vi "Sensor Read 2017.vi"() -> ()   [LabVIEW 2016]
uses:
  Global Variables/Refnum Names.vi
  Global Variables/Sensor Data.vi
panel:
  out "YPR.Yaw":dbl
  out "FusedHeading.Heading":dbl
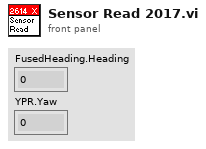
[diagram p1: front panel]
types:
  T1 = typedef "WPI_MotorControlDeviceRef.ctl" = cluster{"DeviceStatus":errorcluster, "Type":T2, "PWM":cluster{"PWM Channel":T3, "DeadBand":T4}, "CAN":cluster{"Device Number":u8, "SetOutput VI Ref":variant, "GetOutput VI Ref":variant, "Enable VI Ref":variant, "Disable VI Ref":variant, "Data":variant}, "Invert":bool}
  T2 = typedef "WPI_MotorControlType.ctl" = enum16{"PWM", "CAN"}
  T3 = typedef "FPGA_DIOPWMChannel.ctl" = enum8{"PWM 0", "PWM 1", "PWM 2", "PWM 3", "PWM 4", "PWM 5", "PWM 6", "PWM 7", "PWM 8", "PWM 9", "PWM MXP 0", "PWM MXP 1", "PWM MXP 2", "PWM MXP 3", "PWM MXP 4", "PWM MXP 5", "PWM MXP 6", "PWM MXP 7", "PWM MXP 8", "PWM MXP 9", "Invalid"}
  T4 = typedef "WPI_PWMDeadband.ctl" = cluster{"Name":string, "maxPositivePwm":i32, "minPositivePwm":i32, "centerPwm":i32, "maxNegativePwm":i32, "minNegativePwm":i32, "angularRange":u16}
  T5 = typedef "CTRE_PigeonIMU_DeviceRef.ctl" = cluster{"DeviceStatus":errorcluster, "Device Number":u8, "Type":T6, "Device ID":u32}
  T6 = typedef "CTRE_PigeonIMU_ConnectionType.ctl" = u32
  T7 = typedef "WPI_DigitalInputDevRef.ctl" = cluster{"DevStatus":errorcluster, "DIO Channel":T8}
  T8 = typedef "FPGA_DIOChannel.ctl" = enum8{"DIO 0", "DIO 1", "DIO 2", "DIO 3", "DIO 4", "DIO 5", "DIO 6", "DIO 7", "DIO 8", "DIO 9", "DIO MXP 0", "DIO MXP 1", "DIO MXP 2", "DIO MXP 3", "DIO MXP 4", "DIO MXP 5", "DIO MXP 6", "DIO MXP 7", "DIO MXP 8", "DIO MXP 9", "DIO MXP 10", "DIO MXP 11", "DIO MXP 12", "DIO MXP 13", "DIO MXP 14", "DIO MXP 15", "SPI Port CS1", "SPI Port CS2", "SPI Port CS3", "SPI Port MISO", "SPI Port MOSI", "Invalid"}
  T9 = typedef "CTRE_PigeonIMU_GlobalStatus.ctl" = cluster{"PigeonState":T10, "FusedHeading":cluster{"Heading":dbl, "Valid?":bool, "Fusing?":bool}, "YPR":cluster{"Yaw":dbl, "Pitch":dbl, "Roll":dbl}, "Compass":cluster{"Heading":dbl, "Magnitude":dbl, "Absolute Heading":dbl}, "Accelerometer":cluster{"Biased":cluster{"X":i16, "Y":i16, "Z":i16, "Norm":i16}, "Angles":cluster{"XZ Tilt":dbl, "YZ Tilt":dbl, "XY Tilt":dbl}}, "Magnetometer":cluster{"Raw":cluster{"X":i16, "Y":i16, "Z":i16}, "Biased":cluster{"X":i16, "Y":i16, "Z":i16}}, "Gyro":cluster{"X":dbl, "Y":dbl, "Z":dbl, "Norm":dbl}, "6D Quaternian":cluster{"W":dbl, "X":dbl, "Y":dbl, "Z":dbl}, "Temp. (C)":dbl, "UpTime":u32, "StartupStatus":cluster{"ResetCount":i32, "ResetFlags":i32, "FirmwareVersion":i32, "HasReset?":bool}, "Calibration":cluster{"CurrentMode":T11, "LastCalError":i32, "CalBooting?":bool}, "CAN Error":errorcluster, "AccumGyro":cluster{"X":dbl, "Y":dbl, "Z":dbl}, "Usage Frame":u32}
  T10 = typedef "CTRE_PigeonIMU_PigeonState.ctl" = enum16{"NoComm", "Initializing", "Ready", "UserCalibration"}
  T11 = typedef "CTRE_PigeonIMU_CalibrationMode.ctl" = u16
  T12 = typedef "WPI_CANTalonSRX_GlobalStatus.ctl" = cluster{"Applied Throttle":dbl, "Module Enabled":bool, "CAN Error":errorcluster, "Closed Loop Error":dbl, "Forward Limit Switch Closed":bool, "Reverse Limit Switch Closed":bool, "Sensor Position":dbl, "Sensor Velocity":dbl, "Current":dbl, "Sticky Fault - Over Temp":bool, "Sticky Fault - Under Voltage":bool, "Sticky Fault - Forward Limit":bool, "Sticky Fault - Reverse Limit":bool, "Sticky Fault - Forward Soft Limit":bool, "Sticky Fault - Reverse Soft Limit":bool, "Brake is Enabled":bool, "Encoder Position":dbl, "Encoder Velocity":dbl, "Encoder Index Count":dbl, "Encoder A Pin State":bool, "Encoder B Pin State":bool, "Encoder Index Pin State":bool, "Analog In":dbl, "Analog In Velocity":dbl, "Temperature (C)":dbl, "Battery Voltage":dbl, "Control 5 Is Supported":bool, "Current Profile Slot Select":dbl, "Pos Div 8":bool, "Vel Div 4":bool, "Pulse Width Position":i32, "Pulse Width Velocity":i32, "Pulse Width Rise To Rise (us)":i32, "Pulse Width Rise To Fall (us)":i32, "Mot Prof Active Is Under Run":bool, "Mot Prof Active Has Under Run":bool, "Mot Prof Active Is Last":bool, "Mot Prof Active Velocity Only":bool, "Mot Prof Active Is Valid":bool, "Mot Prof Buffer Is Full":bool, "Mot Prof Active Profile Slot Select":i32, "Mot Prof NextID":i32, "Mot Prof Count":i32, "Mot Prof Active Velocity":dbl, "Mot Prof Active Position":dbl, "Mot Prof Output Enable":i32, "UsageFrame":u32, "Motion Magic Active Trajectory":cluster{"Velocity":dbl, "Position":dbl}}
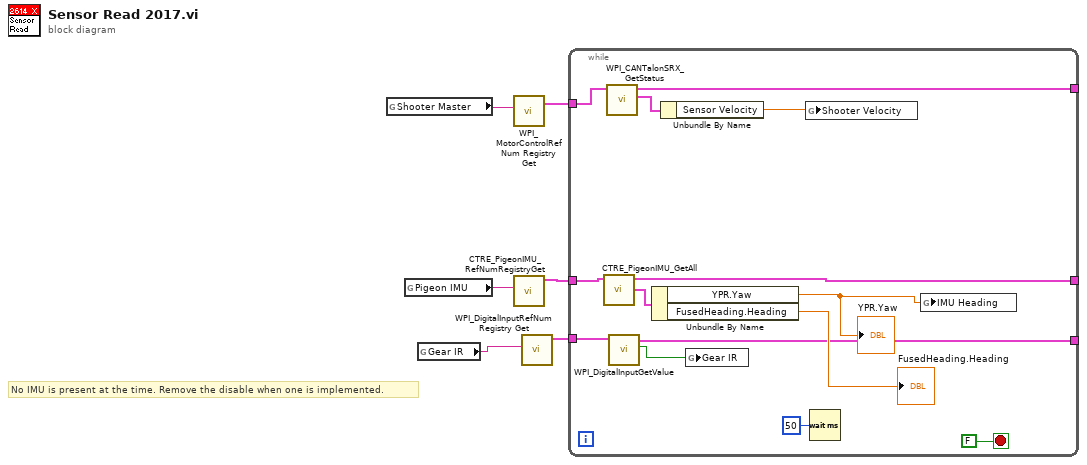
[diagram p0: block diagram]
diagram:
  # "No IMU is present at the time. Remove the disable when one is implemented."
  n1 = global read "Refnum Names.vi" "Shooter Master"() -> (w5:string)
  n2 = global read "Refnum Names.vi" "Pigeon IMU"() -> (w3:string)
  n3 = global read "Refnum Names.vi" "Gear IR"() -> (w2:string)
  n4 = call <vilib>:"WPI_MotorControlRefNum Registry Get.vi"("refnum name"=w5) -> ("MotorControlDevRef"=w6:T1)  [unwired: 9 in, 1 out]
  n5 = call <vilib>:"CTRE_PigeonIMU_RefNumRegistryGet.vi"("refnum name"=w3) -> ("PigeonIMUDevRef"=w4:T5)  [unwired: 9 in, 1 out]
  n6 = call <vilib>:"WPI_DigitalInputRefNum Registry Get.vi"("refnum name"=w2) -> ("DigitalInputDevRef"=w1:T7)  [unwired: 9 in, 1 out]
  n7 = while {
    tunnel: w6 -> [w18]
    tunnel: [w17] -> _
    tunnel: [w16] -> _
    tunnel: w4 -> [w13]
    tunnel: w1 -> [w9]
    tunnel: [w8] -> _
    stop <- FALSE stop-if-true
    n8 = call <vilib>:"CTRE_PigeonIMU_GetAll.vi"("PigeonIMUDevRef"=w13) -> ("Get All"=w12:T9, "PigeonIMUDevRef"=w16:T5)  [unwired: 8 in, 1 out]
    n9 = call <vilib>:"WPI_CANTalonSRX_GetStatus.vi"("CAN Talon SRX Ref"=w18) -> ("Talon SRX Status"=w19:T12, "CAN Talon SRX Ref"=w17:T1)  [unwired: 8 in, 1 out]
    n10 = call <vilib>:"WPI_DigitalInputGetValue.vi"("DigitalInputDevRef"=w9) -> ("Value"=w7:bool, "DigitalInputDevRef"=w8:T7)  [unwired: 8 in, 1 out]
    n11 = Unbundle By Name(w12) -> ("YPR.Yaw"=w11:dbl, "FusedHeading.Heading"=→"FusedHeading.Heading":dbl)
    "YPR.Yaw" <- w11
    n12 = Unbundle By Name(w19) -> ("Sensor Velocity"=w20:dbl)
    n13 = global write "Sensor Data.vi" "Gear IR"(w7) -> ()
    n14 = global write "Sensor Data.vi" "Shooter Velocity"(w20) -> ()
    n15 = Wait (ms)(milliseconds to wait=u32 50) -> ()  [unwired: 1 out]
    n16 = global write "Sensor Data.vi" "IMU Heading"(w11) -> ()
  }
